vi "Measure(old).vi"(8 "error in":errorcluster, 10 "Controle":T2, 11 "map reference in":refnum<data-value>) -> (0 "error out":errorcluster, 2 "Indicator":T2, 3 "map reference out":refnum<data-value>, 4 "Occupancy Grid":dbl[][](graph), 6 "XY Graph":cluster{dbl[], dbl[]}[](graph))   [LabVIEW 2011]
uses:
  <vilib>/robotics/Navigation/shared/WorldMap/OccupancyGridWorldMap/NI_Robotics_OccupancyGridWorldMap.lvclass
panel:
  in  "Lines In":T1(array[cluster]) {"End Point"."Y" format="%.2f"; "End Point"."X" format="%.2f"; "Start Point"."Y" format="%.2f"; "Start Point"."X" format="%.2f"}
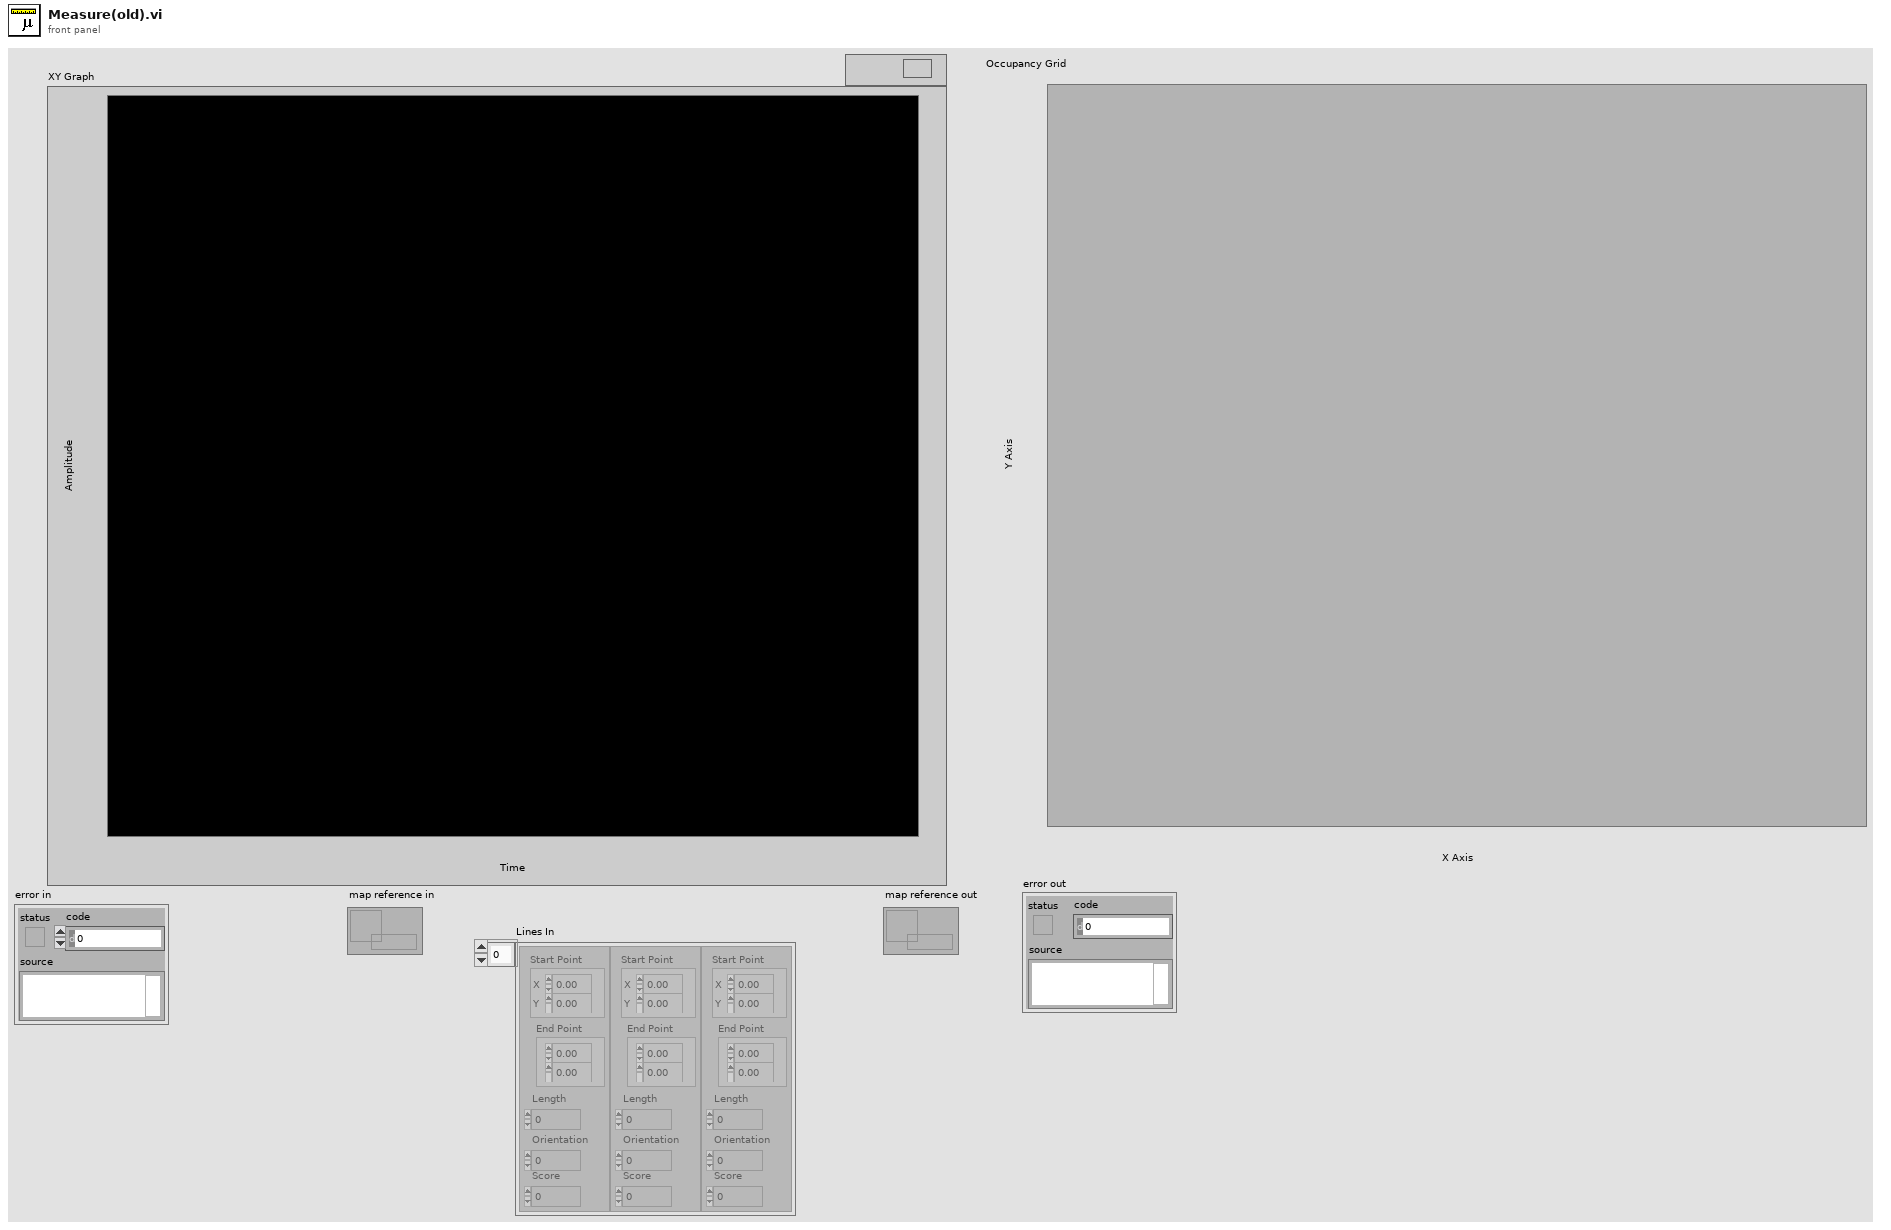
[diagram p1: front panel]
types:
  T1 = cluster{"Start Point":cluster{"X":sgl, "Y":sgl}, "End Point":cluster{"X":sgl, "Y":sgl}, "Length":dbl, "Orientation":dbl, "Score":dbl}[]
  T2 = cluster{"Resolution":i32, "Scale":dbl, "Data":cluster{"GPS Data":cluster{"Latitude":dbl, "Longitude":dbl, "Altitude":dbl, "Velocity, Correction & SET":cluster{"Velocity North":dbl, "Velocity East":dbl, "Velocity Up":dbl, "Ellipsoidal Height":dbl, "GDOP":sgl, "PDOP":sgl, "HDOP":sgl, "VDOP":sgl, "TDOP":sgl, "Horizontal Figure of Merit":u8, "Time Figure of Merit":u8, "Max dGPS Age":sgl, "Extended Navigation Mode":u8, "Antenna Height Adjustment ":dbl, "SET North":i32, "SET East":i32, "SET Up":i32}, "Time":cluster{"GPS Week":u16, "GPS Time of Week":sgl}, "Satellites Used":i32[]}, "IMU Data":cluster{"Position":cluster{"Roll":dbl, "Pitch":dbl, "Yaw":dbl}, "Orientation Matrix":dbl[][], "Magnetic Field":cluster{"Z-Axis Magnetic Field":dbl, "Y-Axis Magnetic Field":dbl, "X-Axis Magnetic Field":dbl}, "Acceleration":cluster{"Z-Axis Acceleration":dbl, "Y-Axis Acceleration":dbl, "X-Axis Acceleration":dbl}, "Angular Rate":cluster{"X-Axis Angular Rate":dbl, "Y-Axis Angular Rate":dbl, "Z-Axis Angular Rate":dbl}, "Quaternion":dbl[]}, "LIDAR Data":cluster{"Magnitude":dbl[], "Direction":dbl[]}, "Telemetry":cluster{"Voltage":cluster{sgl, sgl, sgl}, "Encoder Speed":cluster{i32, i32}, "Temps":cluster{"IC Temp (C)":i32, "Ch1 Temp (C)":i32, "Ch2 Temp (C)":i32}, "Current":cluster{dbl, dbl, dbl, dbl}}, "Lines":cluster{"Start Point":cluster{"X":sgl, "Y":sgl}, "End Point":cluster{"X":sgl, "Y":sgl}, "Length":dbl, "Orientation":dbl, "Score":dbl}[]}, "initialized array":dbl[][]}
  T3 = cluster{"Voltage":cluster{sgl, sgl, sgl}, "Encoder Speed":cluster{i32, i32}, "Temps":cluster{"IC Temp (C)":i32, "Ch1 Temp (C)":i32, "Ch2 Temp (C)":i32}, "Current":cluster{dbl, dbl, dbl, dbl}}
  T4 = cluster{"Latitude":dbl, "Longitude":dbl, "Altitude":dbl, "Velocity, Correction & SET":cluster{"Velocity North":dbl, "Velocity East":dbl, "Velocity Up":dbl, "Ellipsoidal Height":dbl, "GDOP":sgl, "PDOP":sgl, "HDOP":sgl, "VDOP":sgl, "TDOP":sgl, "Horizontal Figure of Merit":u8, "Time Figure of Merit":u8, "Max dGPS Age":sgl, "Extended Navigation Mode":u8, "Antenna Height Adjustment ":dbl, "SET North":i32, "SET East":i32, "SET Up":i32}, "Time":cluster{"GPS Week":u16, "GPS Time of Week":sgl}, "Satellites Used":i32[]}
  T5 = cluster{"Position":cluster{"Roll":dbl, "Pitch":dbl, "Yaw":dbl}, "Orientation Matrix":dbl[][], "Magnetic Field":cluster{"Z-Axis Magnetic Field":dbl, "Y-Axis Magnetic Field":dbl, "X-Axis Magnetic Field":dbl}, "Acceleration":cluster{"Z-Axis Acceleration":dbl, "Y-Axis Acceleration":dbl, "X-Axis Acceleration":dbl}, "Angular Rate":cluster{"X-Axis Angular Rate":dbl, "Y-Axis Angular Rate":dbl, "Z-Axis Angular Rate":dbl}, "Quaternion":dbl[]}
  T6 = cluster{"GPS Data":cluster{"Latitude":dbl, "Longitude":dbl, "Altitude":dbl, "Velocity, Correction & SET":cluster{"Velocity North":dbl, "Velocity East":dbl, "Velocity Up":dbl, "Ellipsoidal Height":dbl, "GDOP":sgl, "PDOP":sgl, "HDOP":sgl, "VDOP":sgl, "TDOP":sgl, "Horizontal Figure of Merit":u8, "Time Figure of Merit":u8, "Max dGPS Age":sgl, "Extended Navigation Mode":u8, "Antenna Height Adjustment ":dbl, "SET North":i32, "SET East":i32, "SET Up":i32}, "Time":cluster{"GPS Week":u16, "GPS Time of Week":sgl}, "Satellites Used":i32[]}, "IMU Data":cluster{"Position":cluster{"Roll":dbl, "Pitch":dbl, "Yaw":dbl}, "Orientation Matrix":dbl[][], "Magnetic Field":cluster{"Z-Axis Magnetic Field":dbl, "Y-Axis Magnetic Field":dbl, "X-Axis Magnetic Field":dbl}, "Acceleration":cluster{"Z-Axis Acceleration":dbl, "Y-Axis Acceleration":dbl, "X-Axis Acceleration":dbl}, "Angular Rate":cluster{"X-Axis Angular Rate":dbl, "Y-Axis Angular Rate":dbl, "Z-Axis Angular Rate":dbl}, "Quaternion":dbl[]}, "LIDAR Data":cluster{"Magnitude":dbl[], "Direction":dbl[]}, "Telemetry":cluster{"Voltage":cluster{sgl, sgl, sgl}, "Encoder Speed":cluster{i32, i32}, "Temps":cluster{"IC Temp (C)":i32, "Ch1 Temp (C)":i32, "Ch2 Temp (C)":i32}, "Current":cluster{dbl, dbl, dbl, dbl}}, "Lines":cluster{"Start Point":cluster{"X":sgl, "Y":sgl}, "End Point":cluster{"X":sgl, "Y":sgl}, "Length":dbl, "Orientation":dbl, "Score":dbl}[]}
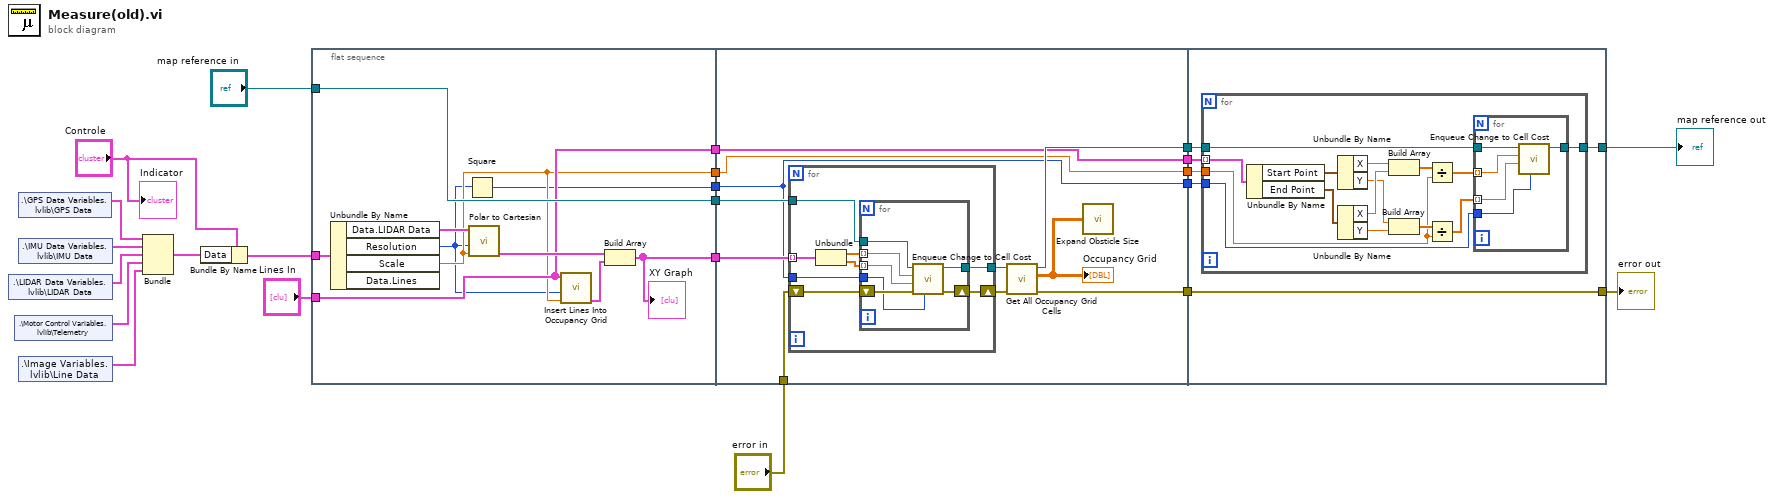
[diagram p0: block diagram]
diagram:
  n1 = shared-variable ".\\LIDAR Data Variables.lvlib\\LIDAR Data"() -> (w17:cluster{"Magnitude":dbl[], "Direction":dbl[]})  [unwired: 1 in, 1 out]
  n2 = shared-variable ".\\Motor Control Variables.lvlib\\Telemetry"() -> (w16:T3)  [unwired: 1 in, 1 out]
  n3 = shared-variable ".\\GPS Data Variables.lvlib\\GPS Data"() -> (w19:T4)  [unwired: 1 in, 1 out]
  n4 = shared-variable ".\\IMU Data Variables.lvlib\\IMU Data"() -> (w18:T5)  [unwired: 1 in, 1 out]
  n5 = shared-variable ".\\Image Variables.lvlib\\Line Data"() -> (w15:T1)  [unwired: 1 in, 1 out]
  n6 = Bundle("GPS Data"=w19, "IMU Data"=w18, "LIDAR Data"=w17, "Telemetry"=w16, "Lines"=w15) -> (w14:T6)  [unwired: 1 in]
  n7 = Bundle By Name(cluster="Controle", "Data"=w14) -> (w13:T2)
  n8 = flat-sequence {
    tunnel: "map reference in" -> [w33]
    tunnel: [w33] -> w20
    tunnel: w13 -> [w32]
    tunnel: "Lines In" -> [w27]
    tunnel: [w28] -> w10
    tunnel: [w27] -> w5
    tunnel: [w26] -> w3
    tunnel: [w24] -> w2
    tunnel: w20 -> [w40]
    tunnel: w10 -> [w43]
    tunnel: "error in" -> [w39]
    tunnel: [w42] -> w8
    tunnel: [w41] -> w7
    tunnel: [w36] -> w6
    tunnel: w5 -> [w36]
    tunnel: [w35] -> w4
    tunnel: w3 -> [w35]
    tunnel: w2 -> [w34]
    tunnel: [w34] -> w1
    tunnel: [w65] -> w22
    tunnel: [w61] -> w23
    tunnel: w8 -> [w62]
    tunnel: w7 -> [w65]
    tunnel: w6 -> [w64]
    tunnel: w4 -> [w63]
    tunnel: w1 -> [w60]
    frame #0 {
      n9 = Unbundle By Name(w32) -> ("Data.LIDAR Data"=w31:cluster{"Magnitude":dbl[], "Direction":dbl[]}, "Resolution"=w25:i32, "Scale"=w26:dbl)  [unwired: 1 out]
      n10 = Square(x=w25) -> (x^2=w24:i32)
      n11 = call "Polar to Cartesian.vi"("Scale"=w26, "Resulotion"=w25, "LIDAR Data"=w31) -> ("XY"=w30:cluster{dbl[], dbl[]})  [unwired: 7 in, 1 out]
      n12 = call "Insert Lines Into Occupancy Grid.vi"("Scale"=w26, "Resolution"=w25, "Lines In"=w27) -> ("XY"=w29:cluster{dbl[], dbl[]})  [unwired: 7 in, 1 out]
      n13 = Build Array(w30, w29) -> (w28:cluster{dbl[], dbl[]}[])
      "XY Graph" <- w28
    }
    frame #1 {
      n14 = for {
        tunnel: [w52] -> w44
        tunnel: w43 -> [w49] mode=indexing
        tunnel: w40 -> [w48]
        shift-right: [w46] -> w38
        shift-left: w39 -> [w47]
        tunnel: w34 -> [w45]
        n15 = Unbundle(w49) -> (w50:dbl[], w51:dbl[])
        n16 = for {
          tunnel: w50 -> [w58] mode=indexing
          tunnel: w51 -> [w59] mode=indexing
          tunnel: w48 -> [w57]
          tunnel: [w56] -> w52
          shift-right: [w54] -> w46
          shift-left: w47 -> [w55]
          tunnel: w45 -> [w53]
          n17 = call <vilib>:"Enqueue Change to Cell Cost.vi"("cost"=w53, "error in (no error)"=w55, "y"=w59, "x"=w58, "map reference in"=w57) -> ("error out"=w54:errorcluster, "map reference out"=w56:refnum<data-value>)  [unwired: 5 in]
        }
      }
      n18 = call <vilib>:"Get All Occupancy Grid Cells.vi"("error in (no error)"=w38, "map reference in"=w44) -> ("error out"=w41:errorcluster, "occupancy grid"=w37:dbl[][], "map reference out"=w42:refnum<data-value>)  [unwired: 7 in]
      "Occupancy Grid" <- w37
      n19 = call "Expand Obsticle Size.vi"("Map In"=w37) -> ()  [unwired: 1 out]
    }
    frame #2 {
      n20 = for {
        tunnel: w64 -> [w80] mode=indexing
        tunnel: w63 -> [w71]
        tunnel: w62 -> [w68]
        tunnel: [w67] -> w61
        tunnel: w60 -> [w66]
        n21 = Unbundle By Name(w80) -> ("Start Point"=w78:cluster{"X":sgl, "Y":sgl}, "End Point"=w79:cluster{"X":sgl, "Y":sgl})
        n22 = Unbundle By Name(w78) -> ("X"=w77:sgl, "Y"=w75:sgl)
        n23 = Unbundle By Name(w79) -> ("X"=w76:sgl, "Y"=w74:sgl)
        n24 = Build Array(w77, w76) -> (w73:sgl[])
        n25 = Build Array(w75, w74) -> (w72:sgl[])
        n26 = Divide(x=w73, y=w71) -> (x/y=w70:dbl[])
        n27 = Divide(x=w72, y=w71) -> (x/y=w69:dbl[])
        n28 = for {
          tunnel: w70 -> [w83] mode=indexing
          tunnel: w69 -> [w82] mode=indexing
          tunnel: w68 -> [w84]
          tunnel: [w85] -> w67
          tunnel: w66 -> [w81]
          n29 = call <vilib>:"Enqueue Change to Cell Cost.vi"("cost"=w81, "y"=w82, "x"=w83, "map reference in"=w84) -> ("map reference out"=w85:refnum<data-value>)  [unwired: 6 in, 1 out]
        }
      }
    }
  }
  "map reference out" <- w23
  "error out" <- w22
  "Indicator" <- "Controle"
